vi "Initialize OOB in Measurement Logic.vi"(8 "error in":errorcluster, 9 "timeout ms (5000)":i32=5000, 10 "retries (10)":i32=10, 11 "OOB Notifier Name":string="OOB gRPC Port") -> (0 "error out":errorcluster, 3 "OBB Port":i32)   [LabVIEW 2025, in "CAN-LIN Raw Bus Capture.lvclass"]
doc: "Connect to the OOB gRPC notifier and acquire the OOB gRPC Listening port to pass to the UI."
uses:
  CAN-LIN Raw Bus Capture.lvclass
  CAN-LIN Raw Bus Capture.lvclass/CAN-LIN Raw Bus Capture.ctl
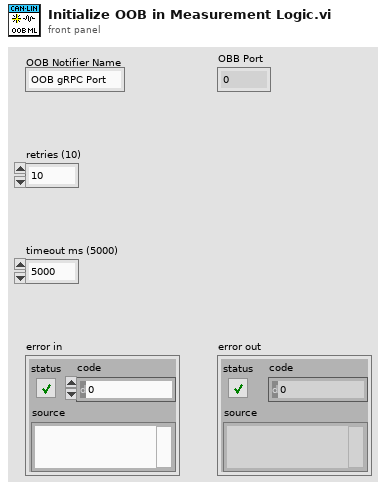
[diagram p1: front panel]
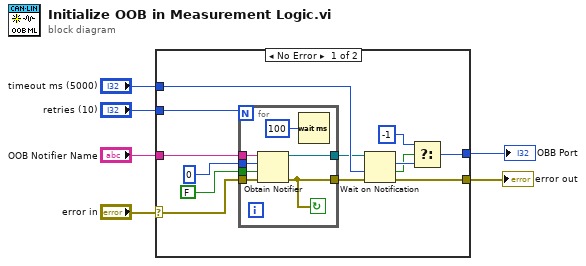
[diagram p0: block diagram]
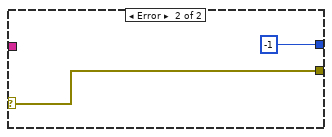
[diagram p2: hidden frame]
diagram:
  n1 = case shown="No Error" "error in" {
    selector: "error in" -> [w7 w28]
    tunnel: [w19 -1 ("i32")] -> w6
    tunnel: "timeout ms (5000)" -> [w17 _]
    tunnel: [w12 w28] -> w4
    tunnel: "OOB Notifier Name" -> [w9 _]
    tunnel: "retries (10)" -> [w8 _]
    frame No Error {
      n2 = for {
        N: w8 -> [_]
        tunnel: [w24] -> w11
        tunnel: [w26] -> w16
        tunnel: w9 -> [w20]
        tunnel: 0 ("i32") -> [w23]
        tunnel: w7 -> [w22]
        tunnel: FALSE ("create if not found?") -> [w21]
        stop <- w24 continue-if-true
        n3 = Obtain Notifier(name (unnamed)=w20, notification data type=w23, create if not found? (T)=w21, error in (no error)=w22) -> (notifier out=w26:refnum<notifier>, error out=w24:errorcluster)  [unwired: 1 out]
        n4 = Wait (ms)(milliseconds to wait=u32 100) -> ()  [unwired: 1 out]
      }
      n5 = Wait on Notification(notifier=w16, timeout in ms (-1)=w17, error in (no error)=w11) -> (notification=w14:i32, timed out?=w13:bool, error out=w12:errorcluster)  [unwired: 1 in, 1 out]
      n6 = Select(t=-1, s=w13, f=w14) -> (s? t:f=w19:i32)
    }
    frame Error {
    }
  }
  "OBB Port" <- w6
  "error out" <- w4
